vi "TCP_Global.vi"() -> ()   [LabVIEW 2015]
panel:
  out "Shutdown":bool
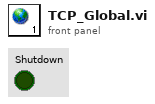
[diagram p1: front panel]
diagram:
